vi "TabCheck.vi"(8 "What I think the tab is":T1) -> (1 "Stop current loop":bool)   [LabVIEW 2010]
uses:
  TabEnum.ctl
  7.0-Global.vi
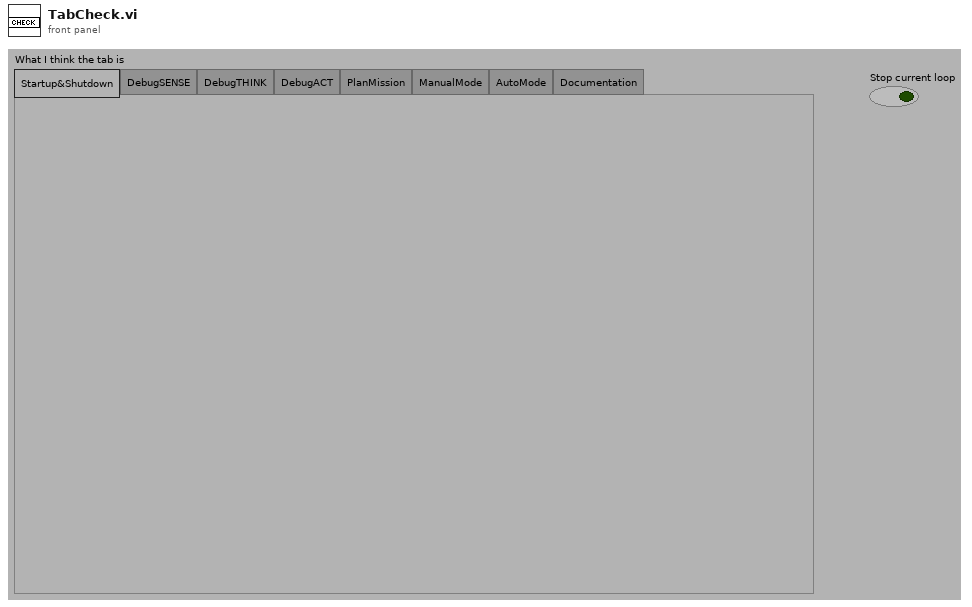
[diagram p1: front panel]
types:
  T1 = typedef "TabEnum.ctl" = enum32{"Startup&Shutdown", "DebugSENSE", "DebugTHINK", "DebugACT", "PlanMission", "ManualMode", "AutoMode", "Documentation"}
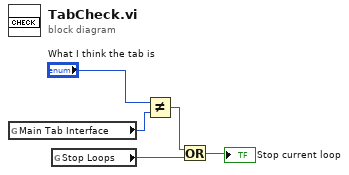
[diagram p0: block diagram]
diagram:
  n1 = global read "7.0-Global.vi" "Main Tab Interface"() -> (w2:T1)
  n2 = global read "7.0-Global.vi" "Stop Loops"() -> (w4:bool)
  n3 = Not Equal?(x="What I think the tab is", y=w2) -> (x != y?=w3:bool)
  n4 = Or(x=w3, y=w4) -> (x .or. y?=→"Stop current loop":bool)
